vi "Application_GetAttributes.vi"(8 "ErrorIn":errorcluster, 10 "OnlyGetDvrReference(False)":bool, 11 "ReferenceIn":refnum<class "Application.lvclass">) -> (0 "ErrorOut":errorcluster, 1 "DataRef":refnum<data-value>, 2 "Data":T1={"Objects"=variant(dbl 0.0), "BasePath"=path "", "Application"=refnum}, 3 "ReferenceOut":refnum<class "Application.lvclass">)   [LabVIEW 2021, in "Application.lvclass"]
uses:
  Application.lvclass
  ObjectAttributes.ctl
  Application.lvclass/Application.ctl
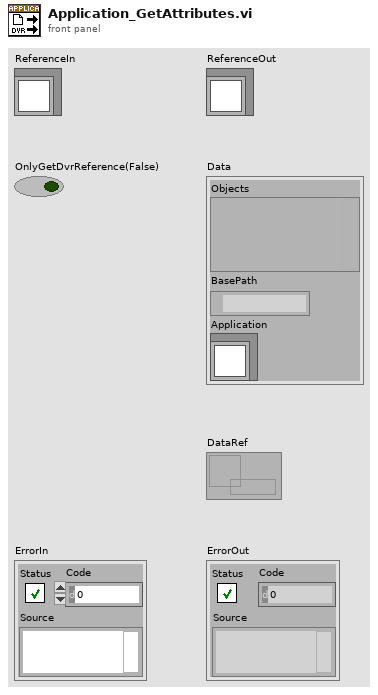
[diagram p1: front panel]
types:
  T1 = typedef "Application.lvclass/ObjectAttributes.ctl" = cluster{"Objects":variant, "BasePath":path, "Application":refnum<class "Application.lvclass">}
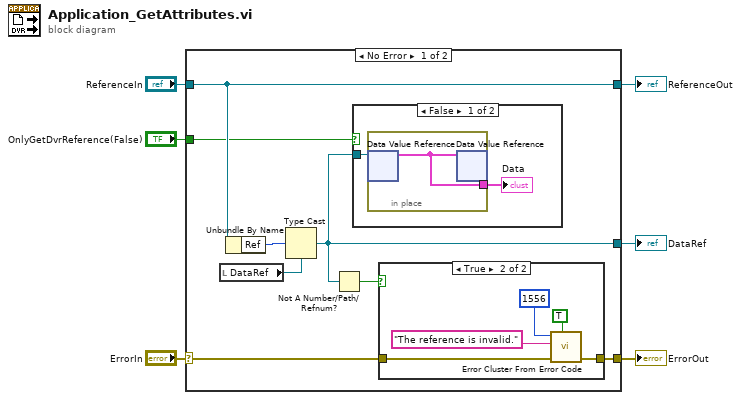
[diagram p0: block diagram]
diagram:
  n1 = case shown="No Error" "ErrorIn" {
    selector: "ErrorIn" -> [w14 w25]
    tunnel: [w13 w25] -> w5
    tunnel: [w12 w24] -> w3
    tunnel: "ReferenceIn" -> [w12 w24]
    tunnel: [w8 _] -> w2
    tunnel: "OnlyGetDvrReference(False)" -> [w9 _]
    frame No Error {
      n2 = local read "DataRef"() -> (w10:refnum<data-value>)
      n3 = Unbundle By Name(w12) -> ("Ref"=w11:u32)
      n4 = Type Cast(type=w10, x=w11) -> (*(type *) &x=w8:refnum<data-value>)
      n5 = Not A Number/Path/Refnum?(number/path/refnum=w8) -> (NaN/Path/Refnum?=w7:bool)
      n6 = case shown="False" w9 {
        tunnel: w8 -> [w22 _]
        frame False {
          n7 = in-place {
            in-place-border: [w23] -> w21
            n8 = in-place-dvr #1(w22) -> (w23:T1)  [unwired: 1 out]
            n9 = in-place-dvr #1(w23) -> ()  [unwired: 2 out]
          }
          "Data" <- w21
        }
        frame True {
        }
      }
      n10 = case shown="True" w7 {
        tunnel: w14 -> [w15 w20]
        tunnel: [w15 w19] -> w13
        frame False {
        }
        frame True {
          n11 = call <vilib>:"Error Cluster From Error Code.vi"("show call chain? (False)"=TRUE, "error in (no error)"=w20, "error message (\"\")"="The reference is invalid." ("source"), "error code (0)"=1556 ("code")) -> ("error out"=w19:errorcluster)  [unwired: 5 in]
        }
      }
    }
    frame Error {
    }
  }
  "ErrorOut" <- w5
  "ReferenceOut" <- w3
  "DataRef" <- w2
